vi "Register Dynamic Events.vi"(8 "error in (no error)":errorcluster, 11 "PaneEventHandler In":refnum<class "PaneEventHandler.lvclass">) -> (0 "error out":errorcluster, 3 "PaneEventHandler Out":refnum<class "PaneEventHandler.lvclass">)   [LabVIEW 2015, in "ActorEvents.lvlib" / "PaneEventHandler.lvclass"]
uses:
  PaneEventHandler.lvclass
  IEventHandler/IEventHandler.lvclass/IEventHandler.ctl
  <vilib>/event_ctls.llb/lveventtype.ctl
  PaneEventHandler.lvclass/PaneEventHandler.ctl
  IEventHandler/Read Registrations.vi
  IEventHandler/IEventHandler.lvclass
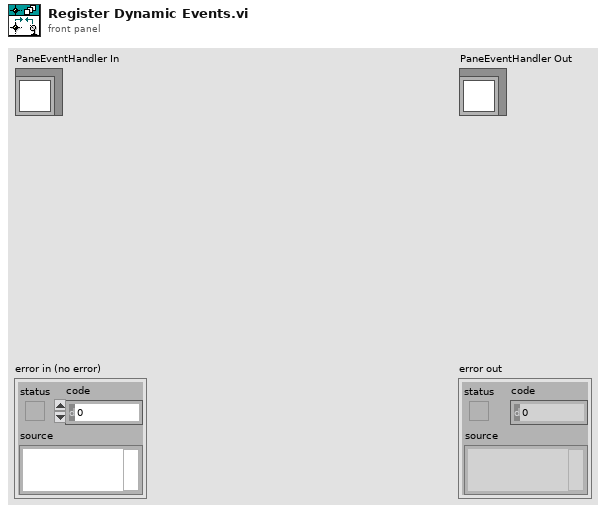
[diagram p1: front panel]
types:
  T1 = typedef "lveventtype.ctl" = enum32{"Null", "Timeout", "Annotation Menu Selection", "Annotation Menu Selection?", "App Instance Close", "App Instance Close?", "Autoscale Range Change", "Bookmark Info Change", "Cell Edit", "Cell Edit?", "Cursor Grab", "Cursor Grab?", "Cursor Menu Selection", "Cursor Menu Selection?", "Cursor Move", "Cursor Release", "Data Change", "Direction Change", "Display State Change", "Drag Ended", "Drag Enter", "Drag Leave", "Drag Over", "Drag Source Update", "Drag Starting", "Drag Starting?", "Drop", "Exec State Change", "Key Down", "Key Down?", "Key Repeat", "Key Repeat?", "Key Up", "Listbox Double Click", "Menu Activation?", "Menu Selection (App)", "Menu Selection? (App)", "Menu Selection (User)", "Mouse Down", "Mouse Down?", "Mouse Enter", "Mouse Leave", "Mouse Move", "Mouse Up", "Mouse Wheel", "NI Security User Change (App)", "Pane Size", "Panel Close", "Panel Close?", "Panel Resize", "Plot Attribute Change", "Scale Range Change", "Shortcut Menu Activation?", "Shortcut Menu Selection (App)", "Shortcut Menu Selection? (App)", "Shortcut Menu Selection (User)", "Tree Double Click", "Tree Drag", "Tree Drag?", "Tree Drop", "Tree Drop?", "Tree Item Close", "Tree Item Close?", "Tree Item Open", "Tree Item Open?", "User Event", "Value Change"}
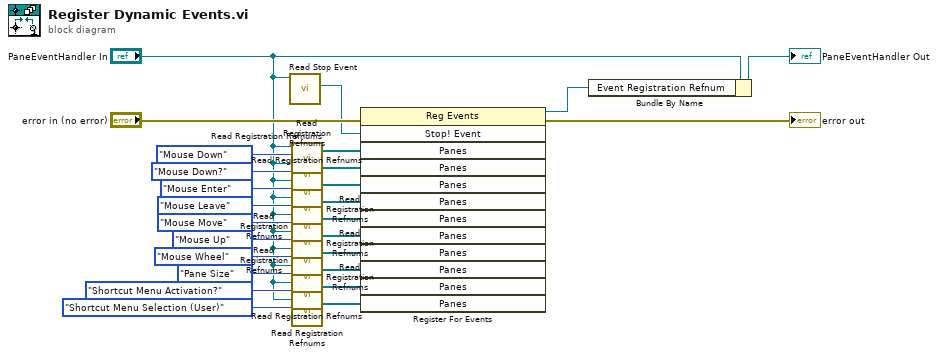
[diagram p0: block diagram]
diagram:
  n1 = call "Read Stop Event.vi"("IEventHandler in"="PaneEventHandler In") -> ("Stop! Event"=w23:refnum<user-event>)  [unwired: 10 in]
  n2 = call "Read Registration Refnums.vi"("Event Type"=lveventtype."Mouse Down", "PaneEventHandler"="PaneEventHandler In") -> ("Panes"=w21:refnum<vi>[])  [unwired: 5 in]
  n3 = call "Read Registration Refnums.vi"("Event Type"=lveventtype."Mouse Down?", "PaneEventHandler"="PaneEventHandler In") -> ("Panes"=w19:refnum<vi>[])  [unwired: 5 in]
  n4 = call "Read Registration Refnums.vi"("Event Type"=lveventtype."Mouse Enter", "PaneEventHandler"="PaneEventHandler In") -> ("Panes"=w18:refnum<vi>[])  [unwired: 5 in]
  n5 = call "Read Registration Refnums.vi"("Event Type"=lveventtype."Mouse Leave", "PaneEventHandler"="PaneEventHandler In") -> ("Panes"=w17:refnum<vi>[])  [unwired: 5 in]
  n6 = call "Read Registration Refnums.vi"("Event Type"=lveventtype."Mouse Move", "PaneEventHandler"="PaneEventHandler In") -> ("Panes"=w16:refnum<vi>[])  [unwired: 5 in]
  n7 = call "Read Registration Refnums.vi"("Event Type"=lveventtype."Mouse Up", "PaneEventHandler"="PaneEventHandler In") -> ("Panes"=w15:refnum<vi>[])  [unwired: 5 in]
  n8 = call "Read Registration Refnums.vi"("Event Type"=lveventtype."Mouse Wheel", "PaneEventHandler"="PaneEventHandler In") -> ("Panes"=w14:refnum<vi>[])  [unwired: 5 in]
  n9 = call "Read Registration Refnums.vi"("Event Type"=lveventtype."Pane Size", "PaneEventHandler"="PaneEventHandler In") -> ("Panes"=w13:refnum<vi>[])  [unwired: 5 in]
  n10 = call "Read Registration Refnums.vi"("Event Type"=lveventtype."Shortcut Menu Activation?", "PaneEventHandler"="PaneEventHandler In") -> ("Panes"=w12:refnum<vi>[])  [unwired: 5 in]
  n11 = call "Read Registration Refnums.vi"("Event Type"=lveventtype."Shortcut Menu Selection (User)", "PaneEventHandler"="PaneEventHandler In") -> ("Panes"=w20:refnum<vi>[])  [unwired: 5 in]
  n12 = register-events(error in="error in (no error)", w23, w21, w19, w18, w17, w16, w15, w14, w13, w12, w20) -> (reference out=w22:refnum<event-registration>, error out=→"error out":errorcluster)  [unwired: 1 in]
  n13 = Bundle By Name(cluster="PaneEventHandler In", "Event Registration Refnum"=w22) -> (→"PaneEventHandler Out":refnum<class "PaneEventHandler.lvclass">)
